vi "WDT Threshold Waveforms DBL.vi"(6 "A Threshold":dbl, 7 "Pre-trigger (s)":dbl, 8 "error in (no error)":errorcluster, 9 "Hammer":waveform(dbl), 11 "Mic":waveform(dbl)) -> (0 "error out":errorcluster, 1 "Hammer out":waveform(dbl), 2 "Triggered?":bool, 3 "Mic out":waveform(dbl))   [LabVIEW 2022 SP3]
panel:
  out "max":dbl
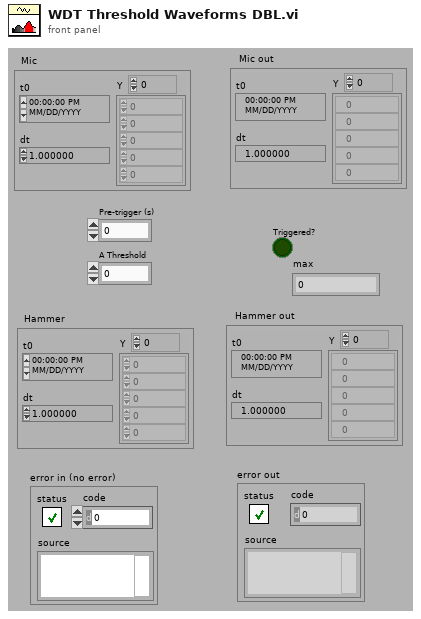
[diagram p1: front panel]
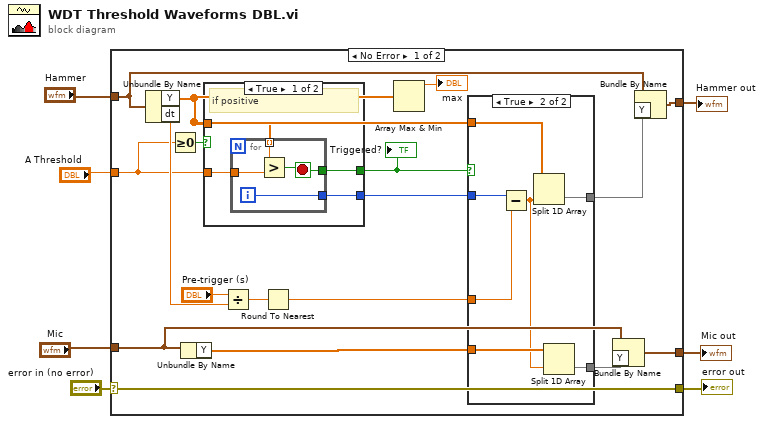
[diagram p0: block diagram]
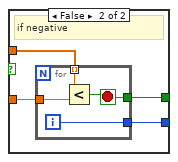
[diagram p2: hidden frame]
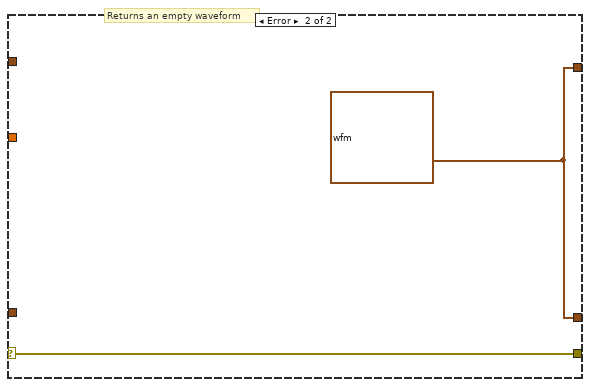
[diagram p4: hidden frame]
diagram:
  n1 = case shown="No Error" "error in (no error)" {
    selector: "error in (no error)" -> [w23 w52]
    tunnel: "Hammer" -> [w25 _]
    tunnel: [w24 w51] -> w1
    tunnel: [w23 w52] -> w6
    tunnel: "A Threshold" -> [w11 _]
    tunnel: "Mic" -> [w16 _]
    tunnel: [w15 w51] -> w2
    frame No Error {
      n2 = Unbundle By Name(w25) -> ("Y"=w9:dbl[], "dt"=w21:dbl)
      n3 = Greater Or Equal To 0?(x=w11) -> (x >= 0?=w10:bool)
      n4 = Unbundle By Name(w16) -> ("Y"=w17:dbl[])
      n5 = case shown="True" w10 {
        tunnel: w11 -> [w29 w37]
        tunnel: w9 -> [w28 w36]
        tunnel: [w27 w35] -> w20
        tunnel: [w26 w34] -> w12
        frame True {
          # "if positive"
          n6 = for {
            tunnel: w28 -> [w33] mode=indexing
            tunnel: w29 -> [w32]
            tunnel: [w31] -> w27
            tunnel: [w30] -> w26
            i -> [w31]
            stop <- w30 stop-if-true
            n7 = Greater?(x=w33, y=w32) -> (0:w30:bool)
          }
        }
        frame False {
          # "if negative"
          n8 = for {
            tunnel: w36 -> [w41] mode=indexing
            tunnel: w37 -> [w40]
            tunnel: [w39] -> w35
            tunnel: [w38] -> w34
            i -> [w39]
            stop <- w38 stop-if-true
            n9 = Less?(x=w41, y=w40) -> (x < y?=w38:bool)
          }
        }
      }
      "Triggered?" <- w12
      n10 = Divide(x="Pre-trigger (s)", y=w21) -> (x/y=w19:dbl)
      n11 = Round To Nearest(number=w19) -> (nearest integer value=w18:dbl)
      n12 = Array Max & Min(array=w9) -> (max value=→"max":dbl)  [unwired: 3 out]
      n13 = case shown="True" w12 {
        tunnel: w9 -> [w43 w50]
        tunnel: w20 -> [_ w49]
        tunnel: w18 -> [_ w48]
        tunnel: w17 -> [w42 w47]
        tunnel: [w42 w45] -> w14
        tunnel: [w43 w44] -> w13
        frame False {
        }
        frame True {
          n14 = Subtract(x=w49, y=w48) -> (x-y=w46:dbl)
          n15 = Split 1D Array(array=w50, index=w46) -> (second subarray=w44:dbl[])  [unwired: 1 out]
          n16 = Split 1D Array(array=w47, index=w46) -> (second subarray=w45:dbl[])  [unwired: 1 out]
        }
      }
      n17 = Bundle By Name(cluster=w16, "Y"=w14) -> (w15:waveform(dbl))
      n18 = Bundle By Name(cluster=w25, "Y"=w13) -> (w24:waveform(dbl))
    }
    frame Error {
      w51 = waveform(dbl) {"t0"=timestamp(0 s since 1904-01-01), "dt"=0.0, "Y"=[]} ("waveform B")
      # "Returns an empty waveform"
      # "Incoming Error"
    }
  }
  "Mic out" <- w2
  "error out" <- w6
  "Hammer out" <- w1
